vi "Read UI Objects.vi"(8 "error in (no error)":errorcluster, 11 "Draw in":refnum<class "Draw.lvclass">) -> (0 "error out":errorcluster, 2 "UI Objects":refnum<class "UI Object.lvclass">[](array[class]), 3 "Draw out":refnum<class "Draw.lvclass">)   [LabVIEW 2016, in "PacManClasses.lvlib" / "Draw.lvclass"]
uses:
  Draw.lvclass
  Geometric Figure/UI Object.lvclass
  Draw.lvclass/Draw.ctl
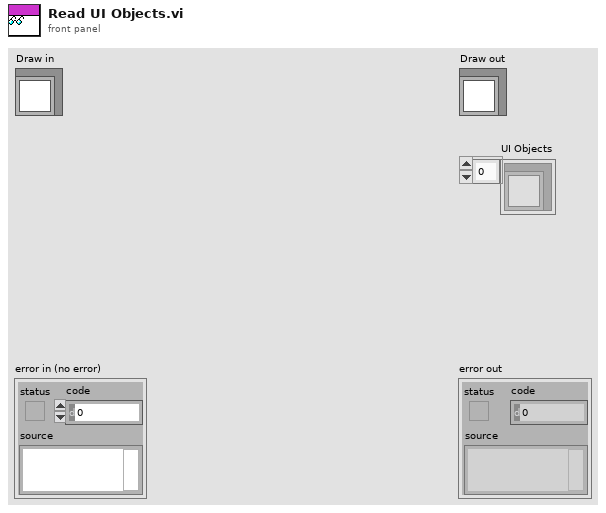
[diagram p1: front panel]
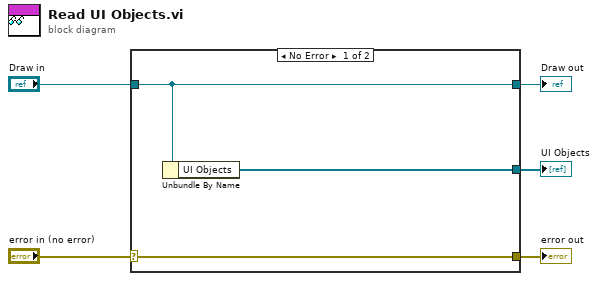
[diagram p0: block diagram]
diagram:
  n1 = case shown="No Error" "error in (no error)" {
    selector: "error in (no error)" -> [w8 w9]
    tunnel: [w8 w9] -> w4
    tunnel: [w7 w10] -> w2
    tunnel: "Draw in" -> [w7 w10]
    tunnel: [w6 _] -> w1
    frame No Error {
      n2 = Unbundle By Name(w7) -> ("UI Objects"=w6:refnum<class "UI Object.lvclass">[])
    }
    frame Error {
    }
  }
  "error out" <- w4
  "Draw out" <- w2
  "UI Objects" <- w1
